vi "Apply Limits.vi"(8 "error in":errorcluster, 11 "PRM in":refnum<class "PRM.lvclass">) -> (0 "error out":errorcluster, 3 "PRM out":refnum<class "PRM.lvclass">)   [LabVIEW 2019, in "PRM.lvlib" / "PRM.lvclass"]
uses:
  Library/PRM.lvclass
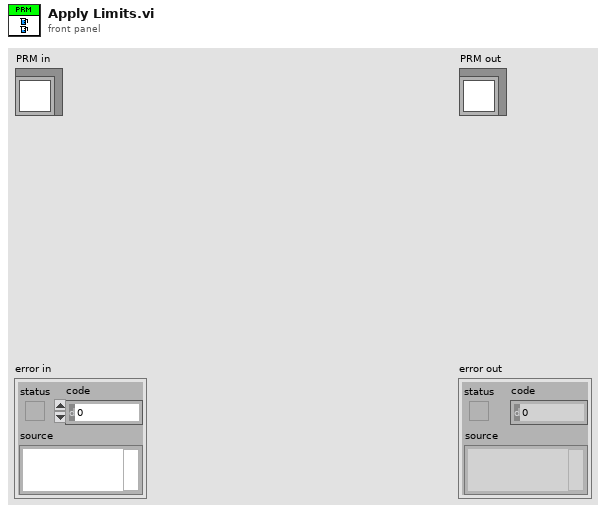
[diagram p1: front panel]
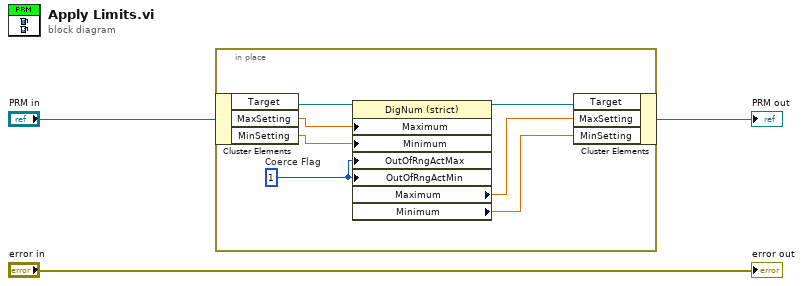
[diagram p0: block diagram]
diagram:
  n1 = in-place {
    w4 = u8 1  # Coerce Flag
    n2 = in-place-cluster #1("PRM in") -> ("Target"=w10:refnum<vi>, "MaxSetting"=w8:dbl, "MinSetting"=w7:dbl)
    n3 = property class="DigNum (strict)"(reference=w10, "Maximum"=w8, "Minimum"=w7, "OutOfRngActMax"=w4, "OutOfRngActMin"=w4) -> (reference out=w9:refnum<vi>, "Maximum"=w6:dbl, "Minimum"=w5:dbl)  [unwired: 1 in, 1 out]
    n4 = in-place-cluster #1("Target"=w9, "MaxSetting"=w6, "MinSetting"=w5) -> (→"PRM out":refnum<class "PRM.lvclass">)
  }
  "error out" <- "error in"
